vi "Add Control Caption.vi"(8 "error in (no error)":errorcluster, 11 "Cluster in":refnum<class "Cluster.lvclass">) -> (0 "error out":errorcluster, 3 "Cluster out":refnum<class "Cluster.lvclass">)   [LabVIEW 2017, in "Localization.lvlib" / "Cluster.lvclass"]
doc: "VI for override that is supposed to do go throgh and create the Caption for the specific VI. Then the caption is set as visible and the label is hidden.\n\nChoose Movement Consulting, LLC"
uses:
  Cluster.lvclass
  C:/Apps/CMC/OpenSource/Localization/Control Info/Control Info.lvclass
  Control Info/Control Info.lvclass
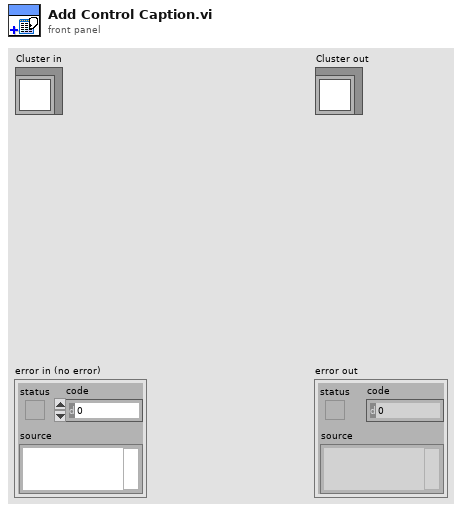
[diagram p1: front panel]
types:
  T1 = typedef "LVPositionTypeDef.ctl" = cluster{"Left":i32, "Top":i32}
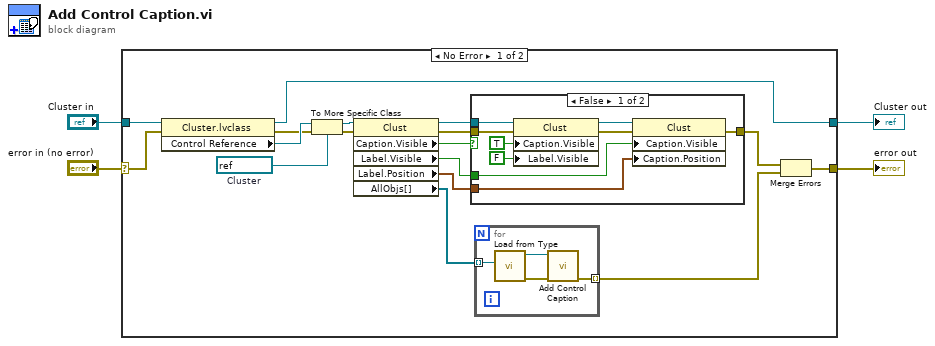
[diagram p0: block diagram]
diagram:
  n1 = case shown="No Error" "error in (no error)" {
    selector: "error in (no error)" -> [w16 w37]
    tunnel: "Cluster in" -> [w15 w36]
    tunnel: [w12 w36] -> w2
    tunnel: [w9 w37] -> w1
    frame No Error {
      w17 = refnum<vi> refnum  # Cluster
      n2 = property class="Cluster.lvclass"(reference=w15, error in=w16) -> (reference out=w12:refnum<class "Cluster.lvclass">, error out=w20:errorcluster, "Control Reference"=w21:refnum<vi>)
      n3 = To More Specific Class(target class=w17, reference=w21, error in=w20) -> (specific class reference=w18:refnum<vi>, error out=w19:errorcluster)
      n4 = property class="Clust"(reference=w18, error in=w19) -> (reference out=w11:refnum<vi>, error out=w13:errorcluster, "Caption.Visible"=w14:bool, "Label.Visible"=w6:bool, "Label.Position"=w5:T1, "AllObjs[]"=w7:refnum<vi>[])
      n5 = case shown="False" w14 {
        tunnel: w13 -> [w33 w35]
        tunnel: w11 -> [w34 _]
        tunnel: [w28 w35] -> w10
        tunnel: w6 -> [w27 _]
        tunnel: w5 -> [w26 _]
        frame False {
          n6 = property class="Clust"(reference=w34, error in=w33, "Caption.Visible"=TRUE, "Label.Visible"=FALSE) -> (reference out=w30:refnum<vi>, error out=w29:errorcluster)
          n7 = property class="Clust"(reference=w30, error in=w29, "Caption.Visible"=w27, "Caption.Position"=w26) -> (error out=w28:errorcluster)  [unwired: 1 out]
        }
        frame True {
        }
      }
      n8 = for {
        tunnel: w7 -> [w25] mode=indexing
        tunnel: [w22] -> w8 mode=indexing
        n9 = call "Load from Type.vi"("Control Reference"=w25) -> ("error out"=w23:errorcluster, "Control Info out"=w24:refnum<class "Control Info.lvclass">)  [unwired: 9 in]
        n10 = call-dynamic "Add Control Caption.vi"("error in (no error)"=w23, "Control Info in"=w24) -> ("error out"=w22:errorcluster)  [unwired: 8 in, 1 out]
      }
      n11 = Merge Errors(w10, w8) -> (w9:errorcluster)
    }
    frame Error {
    }
  }
  "error out" <- w1
  "Cluster out" <- w2
